vi "Sequence.Test.ScanCVX.vi"(7 "Code":T1={"Ready"=FALSE, "DoubleOrder"=FALSE, "OrderDone"=FALSE, "AllowSingleSlot"=FALSE, "CheckDM"=FALSE, "ThresholdA"=0, "ThresholdB"=0, "Plate"=enum."Wabco", "ImgPath"=path "", "Variant"={"State"=enum."Init", "ImgPath"=path "", "WabcoPlate"="", "WabcoProduct"="", "ClientProduct"="", "ClientPlate"="", "TotalQuantity"=0, "OrderQuantity"=0, "Serial"=0, "Wabco"={"LaserJob"="", "AdditionalTxt"="037", "FactoryCode"="", "RevID"=0, "ForkID"=0, "FailuresLimit"=0, "GlobalCnt"=0, "Bank"=0, "SerialFormat"=enum."6 dig", "CoordA"={"X"=0.0, "Y"=0.0, "Angle"=0.0}, "CoordB"={"X"=0.0, "Y"=0.0, "Angle"=0.0}, "DMCconfig"=0}, "Client"={"LaserJob"="", "AdditionalTxt"="", "FactoryCode"="037", "RevID"=0, "ForkID"=0, "FailuresLimit"=0, "GlobalCnt"=0, "Bank"=0, "SerialFormat"=enum."6 dig", "CoordA"={"X"=0.0, "Y"=0.0, "Angle"=0.0}, "CoordB"={"X"=0.0, "Y"=0.0, "Angle"=0.0}, "DMCconfig"=0}}}, 8 "error in":errorcluster, 11 "Data in":T8) -> (0 "error out":errorcluster, 3 "Data out":T8)   [LabVIEW 2016]
uses:
  Station/Station.ProductSlot.ctl
  Sequence.Step.Status.ctl
  Sequence.Prod.StatusData.ctl
  Sequence.Code.Sets.ctl
  Sequence.Slot.StatusData.ctl
  Sequence.Test.Status.ctl
  Sequence.Test.BreakReason.ctl
  Sequence.Test.Unload.Status.ctl
  Logger/Logger.Variant.Sets.ctl
  Station/Station.Changeover.State.vi
  Sequence.Code.SerialFormat.ctl
  Station/Station.Plate.Properties.ctl
  Drivers/V7310/LowLevel/V7310.Job.Sets.ctl
  Sequence.PlateType.ctl
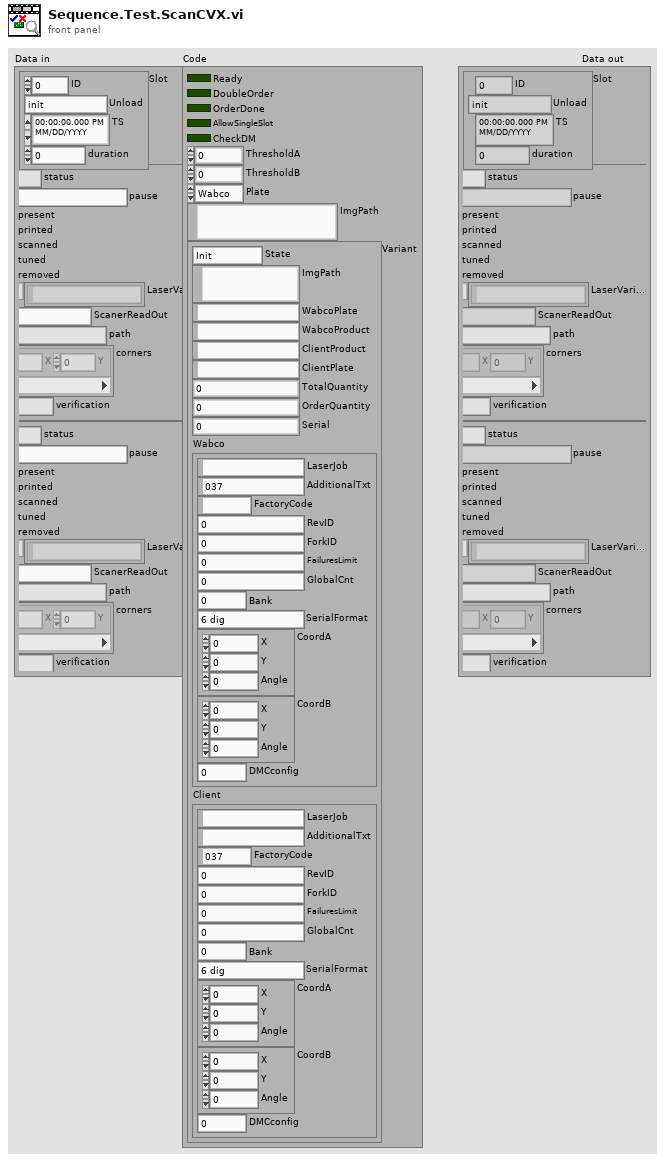
[diagram p1: front panel]
types:
  T1 = typedef "Sequence.Code.Sets.ctl" = cluster{"Ready":bool, "DoubleOrder":bool, "OrderDone":bool, "AllowSingleSlot":bool, "CheckDM":bool, "ThresholdA":u8, "ThresholdB":u8, "Plate":T2, "ImgPath":path, "Variant":T3}
  T2 = typedef "Sequence.PlateType.ctl" = enum16{"Wabco", "Client"}
  T3 = typedef "Logger.Variant.Sets.ctl" = cluster{"State":T4, "ImgPath":path, "WabcoPlate":string, "WabcoProduct":string, "ClientProduct":string, "ClientPlate":string, "TotalQuantity":u16, "OrderQuantity":u16, "Serial":i32, "Wabco":T5, "Client":T5}
  T4 = typedef "Station.Changeover.State.vi" = enum16{"Init", "Scaning", "NOK", "Wait for ack", "Ready"}
  T5 = typedef "Station.Plate.Properties.ctl" = cluster{"LaserJob":string, "AdditionalTxt":string, "FactoryCode":string, "RevID":u8, "ForkID":u8, "FailuresLimit":u16, "GlobalCnt":i32, "Bank":u8, "SerialFormat":T6, "CoordA":T7, "CoordB":T7, "DMCconfig":i32}
  T6 = typedef "Sequence.Code.SerialFormat.ctl" = enum8{"", "6 dig", "7 dig"}
  T7 = typedef "V7310.Job.Sets.ctl" = cluster{"X":dbl, "Y":dbl, "Angle":dbl}
  T8 = typedef "Sequence.Test.Status.ctl" = cluster{"Slot":T9, "A":T11, "B":T11}
  T9 = typedef "Sequence.Slot.StatusData.ctl" = cluster{"ID":i32, "Unload":T10, "TS":timestamp, "duration":u32}
  T10 = typedef "Sequence.Test.Unload.Status.ctl" = enum16{"init", "check NOK", "check OK", "wait on NOK", "wait on OK", "wait on Unload", "done"}
  T11 = typedef "Sequence.Prod.StatusData.ctl" = cluster{"status":T12, "pause":T13, "present":bool, "printed":bool, "scanned":bool, "tuned":bool, "removed":bool, "LaserVariables":string[], "ScanerReadOut":string, "path":path, "corners":cluster{"X":i32, "Y":i32}[], "verification":u8}
  T12 = typedef "Sequence.Step.Status.ctl" = enum16{"-", "Pending", "Running", "Skipped", "Passed", "Failed", "Done", "Error", "Aborted", "Stopped"}
  T13 = typedef "Sequence.Test.BreakReason.ctl" = enum16{"-", "NOK container", "OK container", "Rev empty", "Rev missing", "Rev wrong", "Fork missing", "Fork wrong", "NOK limit", "Unload failure", "Single slot", "Part done", "Err: Prod move work", "Err: Prod move home", "Err: Prod lift work", "Err: Prod lift home", "Err: Prod Arm Work", "Err: Prod Arm NOK", "Err: Prod Arm OK", "Err: Prod NOK suck", "Err: Prod NOK drop", "Err: Prod OK missing", "Err: Prod OK suck", "Err: Prod OK drop"}
  T14 = typedef "Station.ProductSlot.ctl" = enum8{"A", "B"}
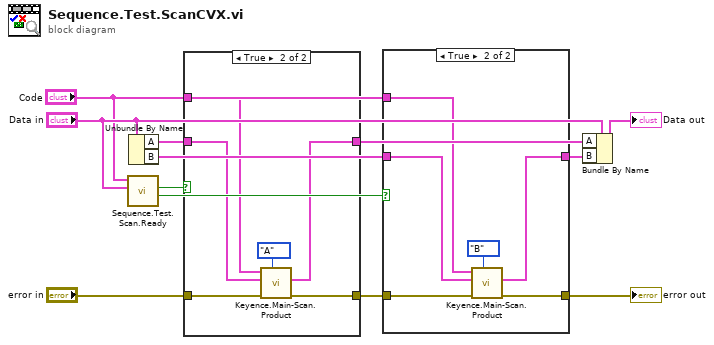
[diagram p0: block diagram]
diagram:
  n1 = call "Sequence.Test.Scan.Ready.vi"("Data in"="Data in", "Code"="Code") -> ("Running B"=w1:bool, "Running A"=w10:bool)  [unwired: 8 in]
  n2 = Unbundle By Name("Data in") -> ("A"=w8:T11, "B"=w5:T11)
  n3 = case shown="True" w10 {
    tunnel: "error in" -> [w14 w20]
    tunnel: [w14 w19] -> w6
    tunnel: "Code" -> [_ w18]
    tunnel: w8 -> [w13 w16]
    tunnel: [w13 w15] -> w7
    frame False {
    }
    frame True {
      n4 = call "Keyence.Main-Scan.Product.vi"("Slot"=Station.ProductSlot."A", "error in"=w20, "Code in"=w16, "Code sets in"=w18) -> ("error out"=w19:errorcluster, "Code out"=w15:T11)  [unwired: 6 in]
    }
  }
  n5 = case shown="True" w1 {
    tunnel: w6 -> [w22 w28]
    tunnel: [w22 w27] -> w3
    tunnel: "Code" -> [_ w26]
    tunnel: w5 -> [w21 w24]
    tunnel: [w21 w23] -> w2
    frame False {
    }
    frame True {
      n6 = call "Keyence.Main-Scan.Product.vi"("Slot"=Station.ProductSlot."B", "error in"=w28, "Code in"=w24, "Code sets in"=w26) -> ("error out"=w27:errorcluster, "Code out"=w23:T11)  [unwired: 6 in]
    }
  }
  "error out" <- w3
  n7 = Bundle By Name(cluster="Data in", "A"=w7, "B"=w2) -> (→"Data out":T8)
